vi "ReferenceMove.vi"(8 "error in (no error)":errorcluster, 10 "Array":dbl[](array[numeric]), 11 "SoftmotionAxis in":refnum<class "SoftmotionAxis.lvclass">) -> (0 "error out":errorcluster, 3 "SoftmotionAxis out":refnum<class "SoftmotionAxis.lvclass">)   [LabVIEW 2017, in "SoftmotionAxis.lvclass"]
uses:
  SoftmotionAxis.lvclass
  <resource>/objmgr/nimotion.rc
  Utilities/WordManipulationLibrary.lvlib
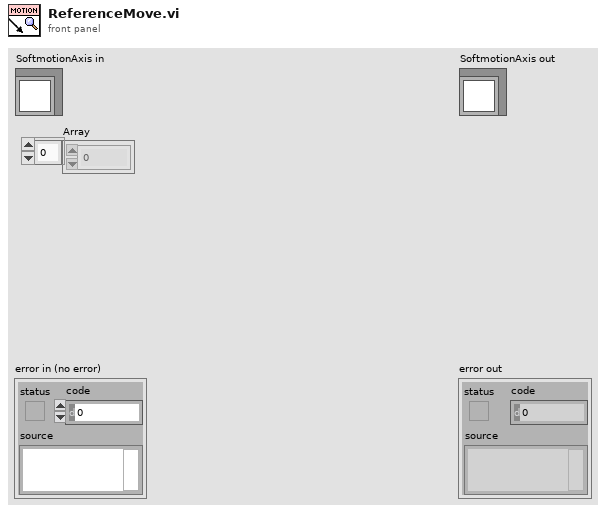
[diagram p1: front panel]
types:
  T1 = typedef "WordManipulationLibrary.lvlib/Parameters_Reference.ctl" = cluster{"Reference Move Mode":i32, "Start Search Forward":bool, "Stop on FWD Edge":bool, "Approach Forward":bool, "Velocity":dbl, "Acceleration":dbl}
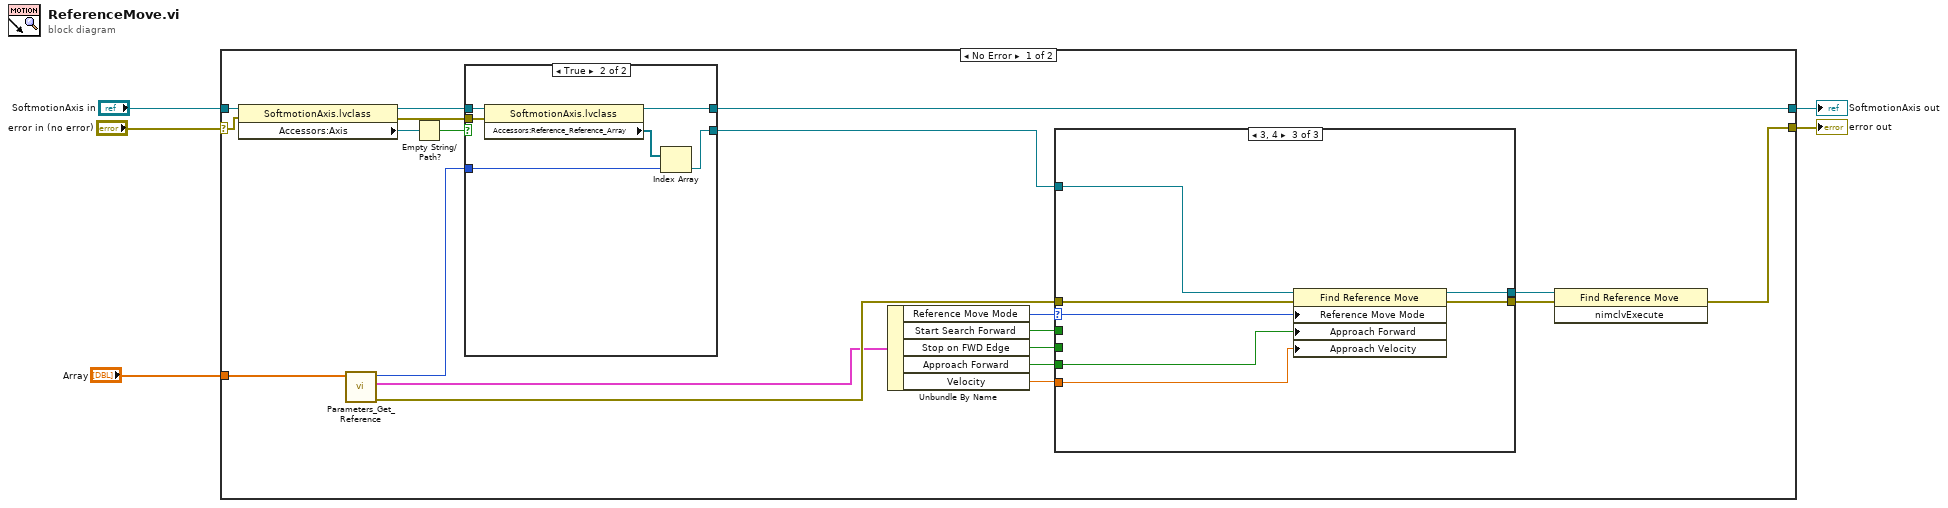
[diagram p0: block diagram]
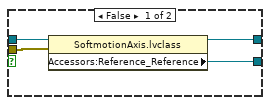
[diagram p2: hidden frame]
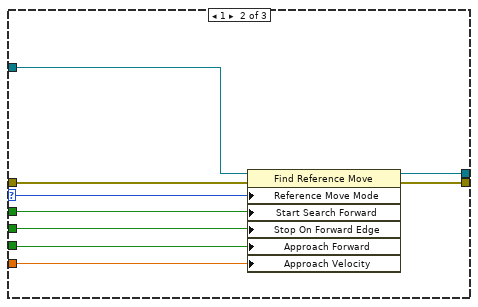
[diagram p4: hidden frame]
diagram:
  n1 = case shown="No Error" "error in (no error)" {
    selector: "error in (no error)" -> [w12 w55]
    tunnel: [w20 w55] -> w4
    tunnel: [w25 w54] -> w2
    tunnel: "SoftmotionAxis in" -> [w13 w54]
    tunnel: "Array" -> [w23 _]
    frame No Error {
      n2 = property class="SoftmotionAxis.lvclass"(reference=w13, error in=w12) -> (reference out=w9:refnum<class "SoftmotionAxis.lvclass">, error out=w8:errorcluster, "Accessors:Axis"=w11:refnum<k21>)
      n3 = call "Parameters_Get_Reference.vi"("Parameters"=w23) -> ("error out"=w15:errorcluster, "Reference Move Parameters"=w7:T1, "Axis to command"=w6:i32)  [unwired: 8 in]
      n4 = Empty String/Path?(string/path=w11) -> (empty?=w10:bool)
      n5 = case shown="True" w10 {
        tunnel: [w29 w34] -> w25
        tunnel: [w28 w31] -> w24
        tunnel: w9 -> [w27 w35]
        tunnel: w8 -> [w26 w33]
        tunnel: w6 -> [_ w30]
        frame False {
          n6 = property class="SoftmotionAxis.lvclass"(reference=w27, error in=w26) -> (reference out=w29:refnum<class "SoftmotionAxis.lvclass">, "Accessors:Reference_Reference"=w28:refnum<k20>)  [unwired: 1 out]
        }
        frame True {
          n7 = property class="SoftmotionAxis.lvclass"(reference=w35, error in=w33) -> (reference out=w34:refnum<class "SoftmotionAxis.lvclass">, "Accessors:Reference_Reference_Array"=w32:refnum<k20>[])  [unwired: 1 out]
          n8 = Index Array(array=w32, index=w30) -> (element=w31:refnum<k20>)
        }
      }
      n9 = Unbundle By Name(w7) -> ("Reference Move Mode"=w19:i32, "Start Search Forward"=w17:bool, "Stop on FWD Edge"=w16:bool, "Approach Forward"=w18:bool, "Velocity"=w14:dbl)
      n10 = case shown="3, 4" w19 {
        selector: w19 -> [_ w40 w48]
        tunnel: w24 -> [w36 w46 w53]
        tunnel: w14 -> [_ w45 w50]
        tunnel: [w36 w44 w52] -> w22
        tunnel: [w37 w43 w51] -> w21
        tunnel: w18 -> [_ w39 w49]
        tunnel: w17 -> [_ w42 _]
        tunnel: w16 -> [_ w41 _]
        tunnel: w15 -> [w37 w38 w47]
        frame 0, Default {
        }
        frame 1 {
          n11 = property class="Find Reference Move"(reference=w46, error in=w38, "Reference Move Mode"=w40, "Start Search Forward"=w42, "Stop On Forward Edge"=w41, "Approach Forward"=w39, "Approach Velocity"=w45) -> (reference out=w44:refnum<k20>, error out=w43:errorcluster)
        }
        frame 3, 4 {
          n12 = property class="Find Reference Move"(reference=w53, error in=w47, "Reference Move Mode"=w48, "Approach Forward"=w49, "Approach Velocity"=w50) -> (reference out=w52:refnum<k20>, error out=w51:errorcluster)
        }
      }
      n13 = invoke class="Find Reference Move" method="nimclvExecute"(reference=w22, error in=w21) -> (error out=w20:errorcluster)  [unwired: 1 in, 2 out]
    }
    frame Error {
    }
  }
  "error out" <- w4
  "SoftmotionAxis out" <- w2
